vi "parse engine statuses.vi"(8 "error in":errorcluster, 11 "message data":string) -> (0 "error out":errorcluster, 3 "value":T1[](array[typedef]))   [LabVIEW 2013, in "module execution process.lvlib"]
uses:
  module execution process.lvlib
  engine status data.ctl
  <vilib>/NI/Module Execution Interface/Engine Runtime/Execution States.ctl
  <vilib>/NI/Module Execution Interface/Engine Runtime/Engine Runtime Interface.lvclass
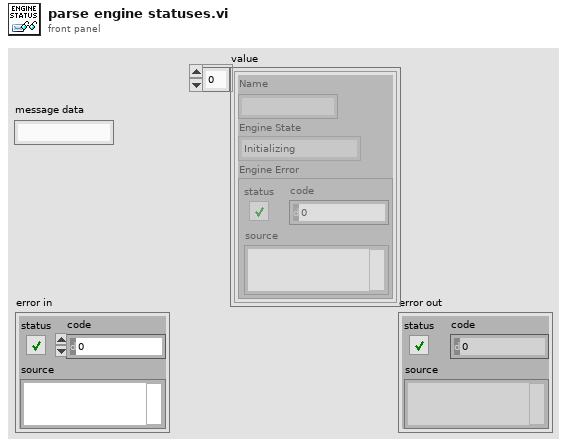
[diagram p1: front panel]
types:
  T1 = typedef "module execution process.lvlib/engine status data.ctl" = cluster{"Name":string, "Engine State":T2, "Engine Error":errorcluster}
  T2 = typedef "Engine Runtime Interface.lvclass/Execution States.ctl" = enum16{"Initializing", "Paused (Initialized)", "Running", "Set Safe Outputs", "Uninitializing", "Stopped (Uninitialized)", "Error (Uninitialized)", "Safe State (Uninitialized)", "Closed"}
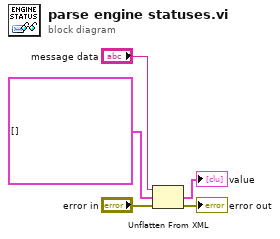
[diagram p0: block diagram]
diagram:
  n1 = Unflatten From XML(xml string="message data", type=T1[] [] ("statuses"), error in (no error)="error in") -> (value=→"value":T1[], error out=→"error out":errorcluster)
